vi "GetImage.vi"(8 "error in (no error)":errorcluster, 10 "Get Image (-1: latest)":i32=-1, 11 "Camera":refnum<class "Camera.lvclass">) -> (0 "error out":errorcluster, 2 "image data":T1, 3 "Camera out":refnum<class "Camera.lvclass">)   [LabVIEW 2015, in "Camera.lvclass"]
doc: "---------------------------------------------------------------\nJKI State Machine Objects™\nhttp://jki.net/state-machine-objects/\nCopyright (C) 2005-2015, JKI <info@jki.net>\nALL RIGHTS RESERVEDJKI State Machine Objects (SMO) 1.0.0.4\nJKI - JKI\nCopyright (c) 2015, JKI"
uses:
  Camera.lvclass
  <vilib>/picture/picture.llb/imagedata.ctl
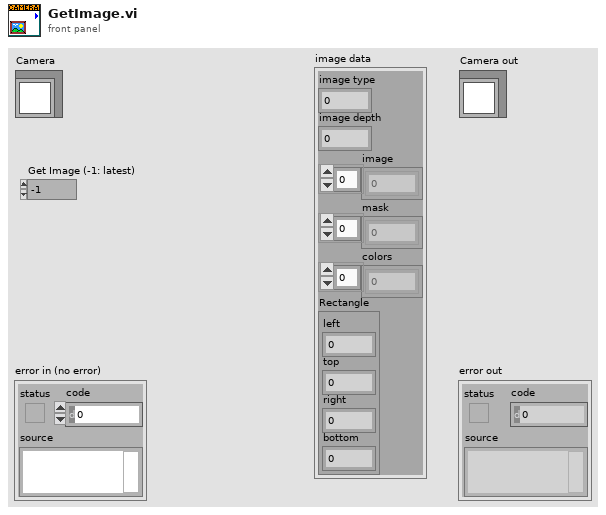
[diagram p1: front panel]
types:
  T1 = typedef "imagedata.ctl" = cluster{"image type":i32, "image depth":i32, "image":u8[], "mask":u8[], "colors":u32[], "Rectangle":cluster{"left":i16, "top":i16, "right":i16, "bottom":i16}}
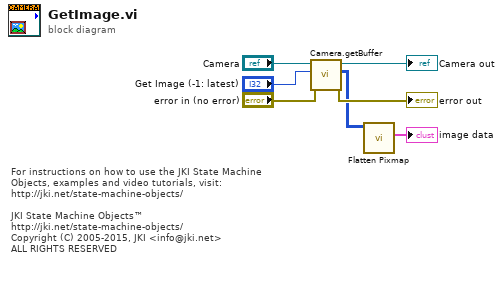
[diagram p0: block diagram]
diagram:
  # "For instructions on how to use the JKI State Machine Objects, examples and video tutorials, visit:\nhttp://jki.net/state-machine-objects/\n\nJKI State Machine Objects™\nhttp://jki.net/state-machine-objects/\nCopyright (C) 2005-2015, JKI <info@jki.net>\nALL RIGHTS RESERVED"
  n1 = call-dynamic "Camera.getBuffer.vi"("error in (no error)"="error in (no error)", "Get Image (-1: latest)"="Get Image (-1: latest)", "Camera in"="Camera") -> ("error out"=→"error out":errorcluster, "pixmap"=w2:u32[][], "Camera out"=→"Camera out":refnum<class "Camera.lvclass">)  [unwired: 6 in]
  n2 = call <vilib>:"Flatten Pixmap.vi"("24-bit pixmap"=w2) -> ("image data"=→"image data":T1)  [unwired: 10 in]
